vi "Send subfolder levels.vi"(8 "error in (no error)":errorcluster, 11 "ImageStack in":refnum<class "Invivo_ImageStack.lvclass">) -> (0 "error out":errorcluster, 3 "ImageStack out":refnum<class "Invivo_ImageStack.lvclass">)   [LabVIEW 2012, in "Invivo_ImageStack.lvclass"]
uses:
  Invivo_ImageStack.lvclass
  <vilib>/Distrio/Murmex/Murmex/update_cluster.ctl
  <vilib>/Distrio/Murmex/Murmex/Murmex.lvclass
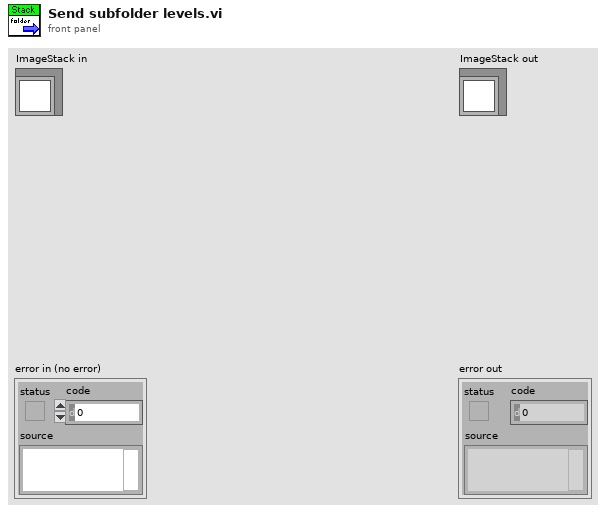
[diagram p1: front panel]
types:
  T1 = typedef "Murmex.lvlib/Murmex.lvclass/update_cluster.ctl" = cluster{"target ID":string, "key chains":string[], "values":variant[]}
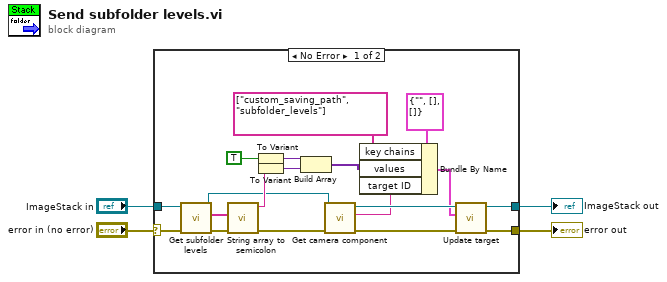
[diagram p0: block diagram]
diagram:
  n1 = case shown="No Error" "error in (no error)" {
    selector: "error in (no error)" -> [w16 w25]
    tunnel: [w23 w25] -> w3
    tunnel: [w19 w24] -> w1
    tunnel: "ImageStack in" -> [w17 w24]
    frame No Error {
      n2 = call-dynamic "Get subfolder levels.vi"("error in (no error)"=w16, "ImageStack in"=w17) -> ("error out"=w15:errorcluster, "Subfolder levels"=w11:string[], "ImageStack out"=w10:refnum<class "Invivo_ImageStack.lvclass">)  [unwired: 7 in]
      n3 = call "String array to semicolon.vi"("error in"=w15, "String array"=w11) -> ("error out"=w14:errorcluster, "Semicolon string"=w13:string)  [unwired: 8 in]
      n4 = To Variant(anything=TRUE) -> (Variant=w5:variant)
      n5 = To Variant(anything=w13) -> (Variant=w12:variant)
      n6 = Build Array(w5, w12) -> (w8:variant[])
      n7 = call-dynamic "Get camera component.vi"("error in (no error)"=w14, "ImageStack in"=w10) -> ("error out"=w21:errorcluster, "Camera component name"=w7:string, "ImageStack out"=w20:refnum<class "Invivo_ImageStack.lvclass">)  [unwired: 7 in]
      n8 = Bundle By Name(cluster=T1 {"target ID"="", "key chains"=[], "values"=[]} ("update cluster"), "key chains"=string[] ["custom_saving_path", "subfolder_levels"], "values"=w8, "target ID"=w7) -> (w9:T1)
      n9 = call <vilib>:"Update target.vi"("error in (no error)"=w21, "update cluster"=w9, "MurmexBase in"=w20) -> ("error out"=w23:errorcluster, "MurmexBase out"=w19:refnum<class "Invivo_ImageStack.lvclass">)  [unwired: 7 in]
    }
    frame Error {
    }
  }
  "error out" <- w3
  "ImageStack out" <- w1
